vi "busy handler.vi"(8 "error in (no error)":errorcluster, 9 "para2":u32, 10 "para1":i32, 11 "para0":dbl) -> (0 "error out":errorcluster, 1 "para2 out":u32, 2 "para1 out":i32, 3 "para0 out":dbl, 5 "function return":i32)   [LabVIEW 2020, in "sqlite3.lvlib"]
uses:
  sqlite3.lvlib
  errstr.vi
  bin/sqlite3_64.dll
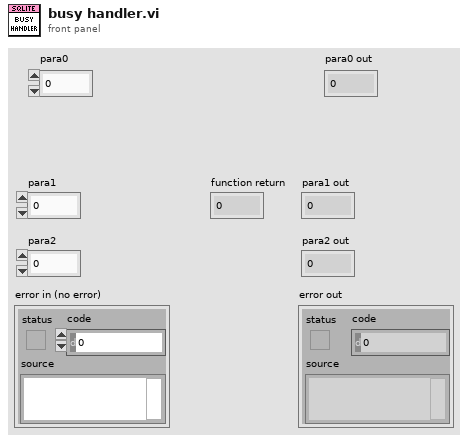
[diagram p1: front panel]
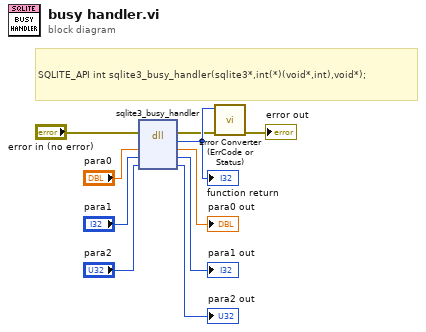
[diagram p0: block diagram]
diagram:
  # "SQLITE_API int sqlite3_busy_handler(sqlite3*,int(*)(void*,int),void*);"
  n1 = dll-call lib="C:/Users/Fred.Guo/Desktop/Database-configuration/externals/sqlite3/Source/bin/sqlite3_*.*" fn="sqlite3_busy_handler"(error in="error in (no error)", "para0"="para0", "para1"="para1", "para2"="para2") -> (error out=w2:errorcluster, w10:i32, "para0"=→"para0 out":dbl, "para1"=→"para1 out":i32, "para2"=→"para2 out":u32)  [unwired: 2 in, 1 out]
  "function return" <- w10
  n2 = call "Error Converter (ErrCode or Status).vi"("error in (no error)"=w2, "error code"=w10) -> ("error out"=→"error out":errorcluster)  [unwired: 9 in]
